vi "Write Pump.vi"(8 "error in":errorcluster, 11 "Pump state":bool=TRUE) -> (0 "error out":errorcluster)   [LabVIEW 2016, in "DAQ.lvlib"]
uses:
  DAQ.lvlib
  support/Message Queue/Message Queue.lvlib
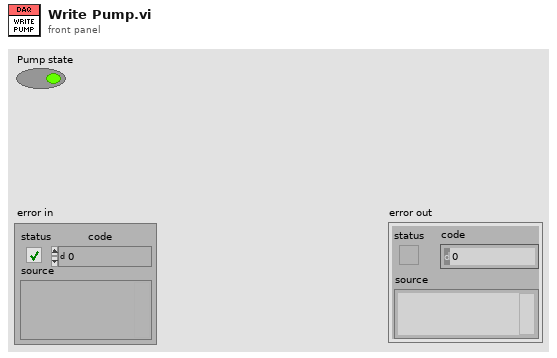
[diagram p1: front panel]
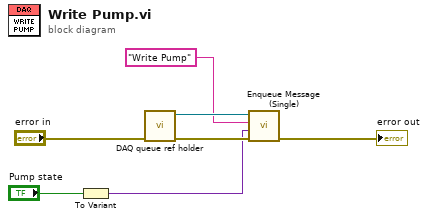
[diagram p0: block diagram]
diagram:
  n1 = To Variant(anything="Pump state") -> (Variant=w1:variant)
  n2 = call "DAQ queue ref holder.vi"("error in"="error in") -> ("error out"=w7:errorcluster, "Input Message Queue"=w4:refnum<queue>)  [unwired: 9 in]
  n3 = call "Enqueue Message (Single).vi"("error in (no error)"=w7, "Message Data"=w1, "Message"="Write Pump", "Message Queue"=w4) -> ("error out"=→"error out":errorcluster)  [unwired: 6 in, 1 out]
